vi "hood.vi"() -> ()   [LabVIEW 2020]
uses:
  TitanLib/Lib/TitanLib.lvlib
  <vilib>/Rock Robotics/WPI/ThirdParty/REV Robotics/REVLib/Typedef/Spark MAX Control Type.ctl
  <vilib>/Rock Robotics/WPI/ThirdParty/Phoenix-LabVIEW/Motor Controller/Controls/CTRE_Phoenix_MotorControl_ControlMode.ctl
panel:
  out "Sensor Position":dbl
  in  "Zero Hood":bool
  in  "Hood Setpoint (deg)":dbl
  in  "Enable Hood":bool
  in  "CTRE Hood Constants":T1
  in  "Max Velocity":dbl
  in  "REV PID Constants":T2={"P Gain"=0.0, "I Gain"=0.0, "D Gain"=0.0, "F Gain"=0.0, "I Zone"=0.0, "Min Output"=-1.0, "Max Output"=1.0}
  in  "Max Acceleration":dbl
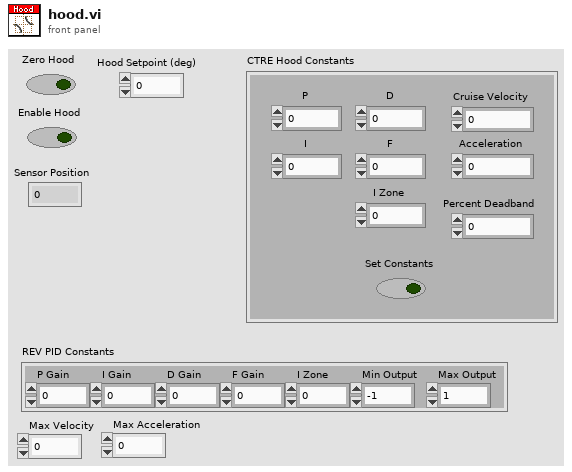
[diagram p1: front panel]
types:
  T1 = cluster{"Set Constants":bool, "P":dbl, "I":dbl, "D":dbl, "F":dbl, "I Zone":dbl, "Cruise Velocity":i32, "Acceleration":i32, "Percent Deadband":dbl}
  T2 = cluster{"P Gain":dbl, "I Gain":dbl, "D Gain":dbl, "F Gain":dbl, "I Zone":dbl, "Min Output":dbl, "Max Output":dbl}
  T3 = typedef "Spark MAX Control Type.ctl" = enum16{"Percent VBus", "Voltage", "Velocity", "Position", "Smart Motion", "Current", "Smart Velocity"}
  T4 = typedef "WPI_MotorControlDeviceRef.ctl" = cluster{"DeviceStatus":errorcluster, "Type":T5, "PWM":cluster{"PWM Channel":T6, "DeadBand":T7}, "CAN":cluster{"Device Number":u8, "SetOutput VI Ref":variant, "GetOutput VI Ref":variant, "Enable VI Ref":variant, "Disable VI Ref":variant, "Data":variant}, "Invert":bool, "DIO PWM":cluster{"PWM \"Enable\" Channel":T6, "DIOChannel":T8, "PWM Rate":dbl}}
  T5 = typedef "WPI_MotorControlType.ctl" = enum16{"PWM", "CAN", "DIO PWM"}
  T6 = typedef "FPGA_DIOPWMChannel.ctl" = enum8{"PWM 0", "PWM 1", "PWM 2", "PWM 3", "PWM 4", "PWM 5", "PWM 6", "PWM 7", "PWM 8", "PWM 9", "PWM MXP 0", "PWM MXP 1", "PWM MXP 2", "PWM MXP 3", "PWM MXP 4", "PWM MXP 5", "PWM MXP 6", "PWM MXP 7", "PWM MXP 8", "PWM MXP 9", "Invalid"}
  T7 = typedef "WPI_PWMDeadband.ctl" = cluster{"Name":string, "maxPositivePwm":i32, "minPositivePwm":i32, "centerPwm":i32, "maxNegativePwm":i32, "minNegativePwm":i32, "angularRange":u16}
  T8 = typedef "FPGA_DIOChannel.ctl" = enum8{"DIO 0", "DIO 1", "DIO 2", "DIO 3", "DIO 4", "DIO 5", "DIO 6", "DIO 7", "DIO 8", "DIO 9", "DIO MXP 0", "DIO MXP 1", "DIO MXP 2", "DIO MXP 3", "DIO MXP 4", "DIO MXP 5", "DIO MXP 6", "DIO MXP 7", "DIO MXP 8", "DIO MXP 9", "DIO MXP 10", "DIO MXP 11", "DIO MXP 12", "DIO MXP 13", "DIO MXP 14", "DIO MXP 15", "SPI Port CS1", "SPI Port CS2", "SPI Port CS3", "SPI Port MISO", "SPI Port MOSI", "Invalid"}
  T9 = typedef "CTRE_Phoenix_MotorControl_ControlMode.ctl" = u16
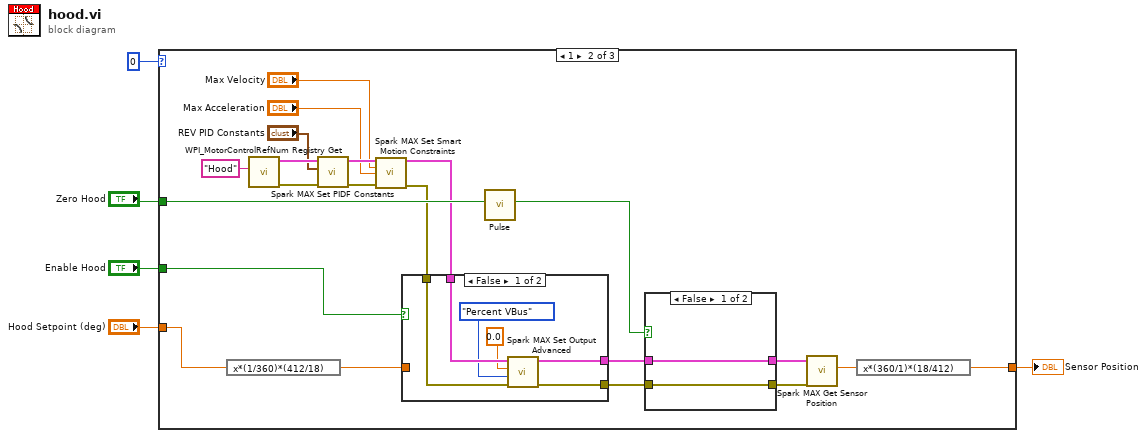
[diagram p0: block diagram]
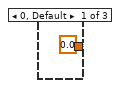
[diagram p2: hidden frame]
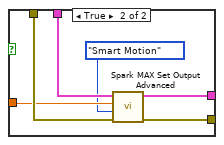
[diagram p3: hidden frame]
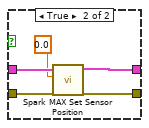
[diagram p4: hidden frame]
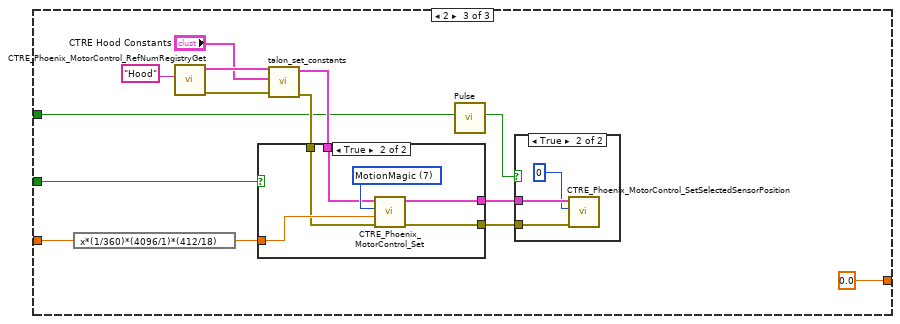
[diagram p5: hidden frame]
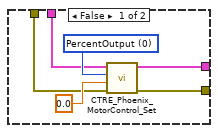
[diagram p6: hidden frame]
diagram:
  n1 = case shown="1" 0 {
    tunnel: "Zero Hood" -> [_ w23 w48]
    tunnel: "Enable Hood" -> [_ w18 w53]
    tunnel: [0.0 ("Sensor Position") w12 0.0 ("Sensor Position")] -> w2
    tunnel: "Hood Setpoint (deg)" -> [_ w15 w51]
    frame 0, Default {
    }
    frame 1 {
      n2 = expression code="x*(1/360)*(412/18)"(w15) -> (w14:dbl)
      n3 = call <vilib>:"WPI_MotorControlRefNum Registry Get.vi"("refnum name"="Hood") -> ("error out"=w26:errorcluster, "MotorControlDevRef"=w25:T4)  [unwired: 9 in]
      n4 = call <vilib>:"Spark MAX Set PIDF Constants.vi"("error in"=w26, "PID Constants"="REV PID Constants", "MotorControlDeviceRef"=w25) -> ("error out"=w10:errorcluster, "MotorControlDeviceRef"=w11:T4)  [unwired: 7 in]
      n5 = call <vilib>:"Spark MAX Set Smart Motion Constraints.vi"("MotorControlDeviceRef"=w11, "Max Velocity"="Max Velocity", "Max Acceleration"="Max Acceleration", "error in"=w10) -> ("MotorControlDeviceRef"=w22:T4, "error out"=w21:errorcluster)  [unwired: 10 in]
      n6 = case shown="False" w18 {
        tunnel: w22 -> [w33 w39]
        tunnel: w21 -> [w32 w38]
        tunnel: [w29 w37] -> w20
        tunnel: [w28 w36] -> w19
        tunnel: w14 -> [_ w35]
        frame False {
          n7 = call <vilib>:"Spark MAX Set Output Advanced.vi"("error in (no error)"=w32, "Control Mode"=Spark_MAX_Control_Type."Percent VBus", "Setpoint"=0.0, "MotorControlDevRef"=w33) -> ("error out"=w28:errorcluster, "MotorControlDevRef"=w29:T4)  [unwired: 6 in]
        }
        frame True {
          n8 = call <vilib>:"Spark MAX Set Output Advanced.vi"("error in (no error)"=w38, "Control Mode"=Spark_MAX_Control_Type."Smart Motion", "Setpoint"=w35, "MotorControlDevRef"=w39) -> ("error out"=w36:errorcluster, "MotorControlDevRef"=w37:T4)  [unwired: 6 in]
        }
      }
      n9 = call "Pulse.vi"("Input"=w23) -> ("Output"=w24:bool)  [unwired: 10 in]
      n10 = case shown="False" w24 {
        tunnel: w20 -> [w41 w46]
        tunnel: w19 -> [w40 w45]
        tunnel: [w41 w43] -> w17
        tunnel: [w40 w42] -> w16
        frame False {
        }
        frame True {
          n11 = call <vilib>:"Spark MAX Set Sensor Position.vi"("error in"=w45, "Position"=0.0, "MotorControlDeviceRef"=w46) -> ("error out"=w42:errorcluster, "MotorControlDeviceRef"=w43:T4)  [unwired: 7 in]
        }
      }
      n12 = call <vilib>:"Spark MAX Get Sensor Position.vi"("error in (no error)"=w16, "MotorControlDevRef in"=w17) -> ("Sensor Position"=w13:dbl)  [unwired: 6 in, 3 out]
      n13 = expression code="x*(360/1)*(18/412)"(w13) -> (w12:dbl)
    }
    frame 2 {
      n14 = expression code="x*(1/360)*(4096/1)*(412/18)"(w51) -> (w50:dbl)
      n15 = call <vilib>:"CTRE_Phoenix_MotorControl_RefNumRegistryGet.vi"("refnum name"="Hood") -> ("error out"=w58:errorcluster, "PhoenixMotorControlDevRef"=w59:T4)  [unwired: 9 in]
      n16 = call "talon_set_constants.vi"("error in"=w58, "Constants"="CTRE Hood Constants", "PhoenixMotorControlDevRef"=w59) -> ("error out"=w55:errorcluster, "PhoenixMotorControlDevRef"=w54:T4)  [unwired: 7 in]
      n17 = case shown="True" w53 {
        tunnel: [w62 w71] -> w57
        tunnel: [w61 w70] -> w56
        tunnel: w50 -> [_ w69]
        tunnel: w55 -> [w63 w68]
        tunnel: w54 -> [w64 w67]
        frame False {
          w66 = T9 0 items=["PercentOutput"=0, "Position"=1, "Velocity"=2, "Current"=3, "Follower"=5, "MotionProfile"=6, "MotionMagic"=7, "MotionProfileArc"=10, "Disabled"=15] ("Control Mode")
          n18 = call <vilib>:"CTRE_Phoenix_MotorControl_Set.vi"("error in (no error)"=w63, "Output"=0.0, "Control Mode"=w66, "PhoenixMotorControlDevRef"=w64) -> ("error out"=w61:errorcluster, "PhoenixMotorControlDevRef"=w62:T4)  [unwired: 6 in]
        }
        frame True {
          w72 = T9 7 items=["PercentOutput"=0, "Position"=1, "Velocity"=2, "Current"=3, "Follower"=5, "MotionProfile"=6, "MotionMagic"=7, "MotionProfileArc"=10, "Disabled"=15] ("Control Mode")
          n19 = call <vilib>:"CTRE_Phoenix_MotorControl_Set.vi"("error in (no error)"=w68, "Output"=w69, "Control Mode"=w72, "PhoenixMotorControlDevRef"=w67) -> ("error out"=w70:errorcluster, "PhoenixMotorControlDevRef"=w71:T4)  [unwired: 6 in]
        }
      }
      n20 = call "Pulse.vi"("Input"=w48) -> ("Output"=w47:bool)  [unwired: 10 in]
      n21 = case shown="True" w47 {
        tunnel: w57 -> [_ w75]
        tunnel: w56 -> [_ w74]
        frame False {
        }
        frame True {
          n22 = call <vilib>:"CTRE_Phoenix_MotorControl_SetSelectedSensorPosition.vi"("error in (no error)"=w74, "New Sensor Position"=0, "PhoenixMotorControlDevRef"=w75) -> ()  [unwired: 7 in, 2 out]
        }
      }
    }
  }
  "Sensor Position" <- w2
